vi "Normal mode logic.vi"(9 "Elevator states array":T1[](array[typedef]), 11 "Floors to serve":cluster{"H call":dbl, "Up":bool}[](array[cluster])) -> (1 "Elevator states array out":T1[](array[typedef]), 3 "Floors to serve out":cluster{"H call":dbl, "Up":bool}[](array[cluster]))   [LabVIEW 2019]
uses:
  Type defs/Elevator states.ctl
  Type defs/Elevator position.ctl
  Type defs/Car buttons.ctl
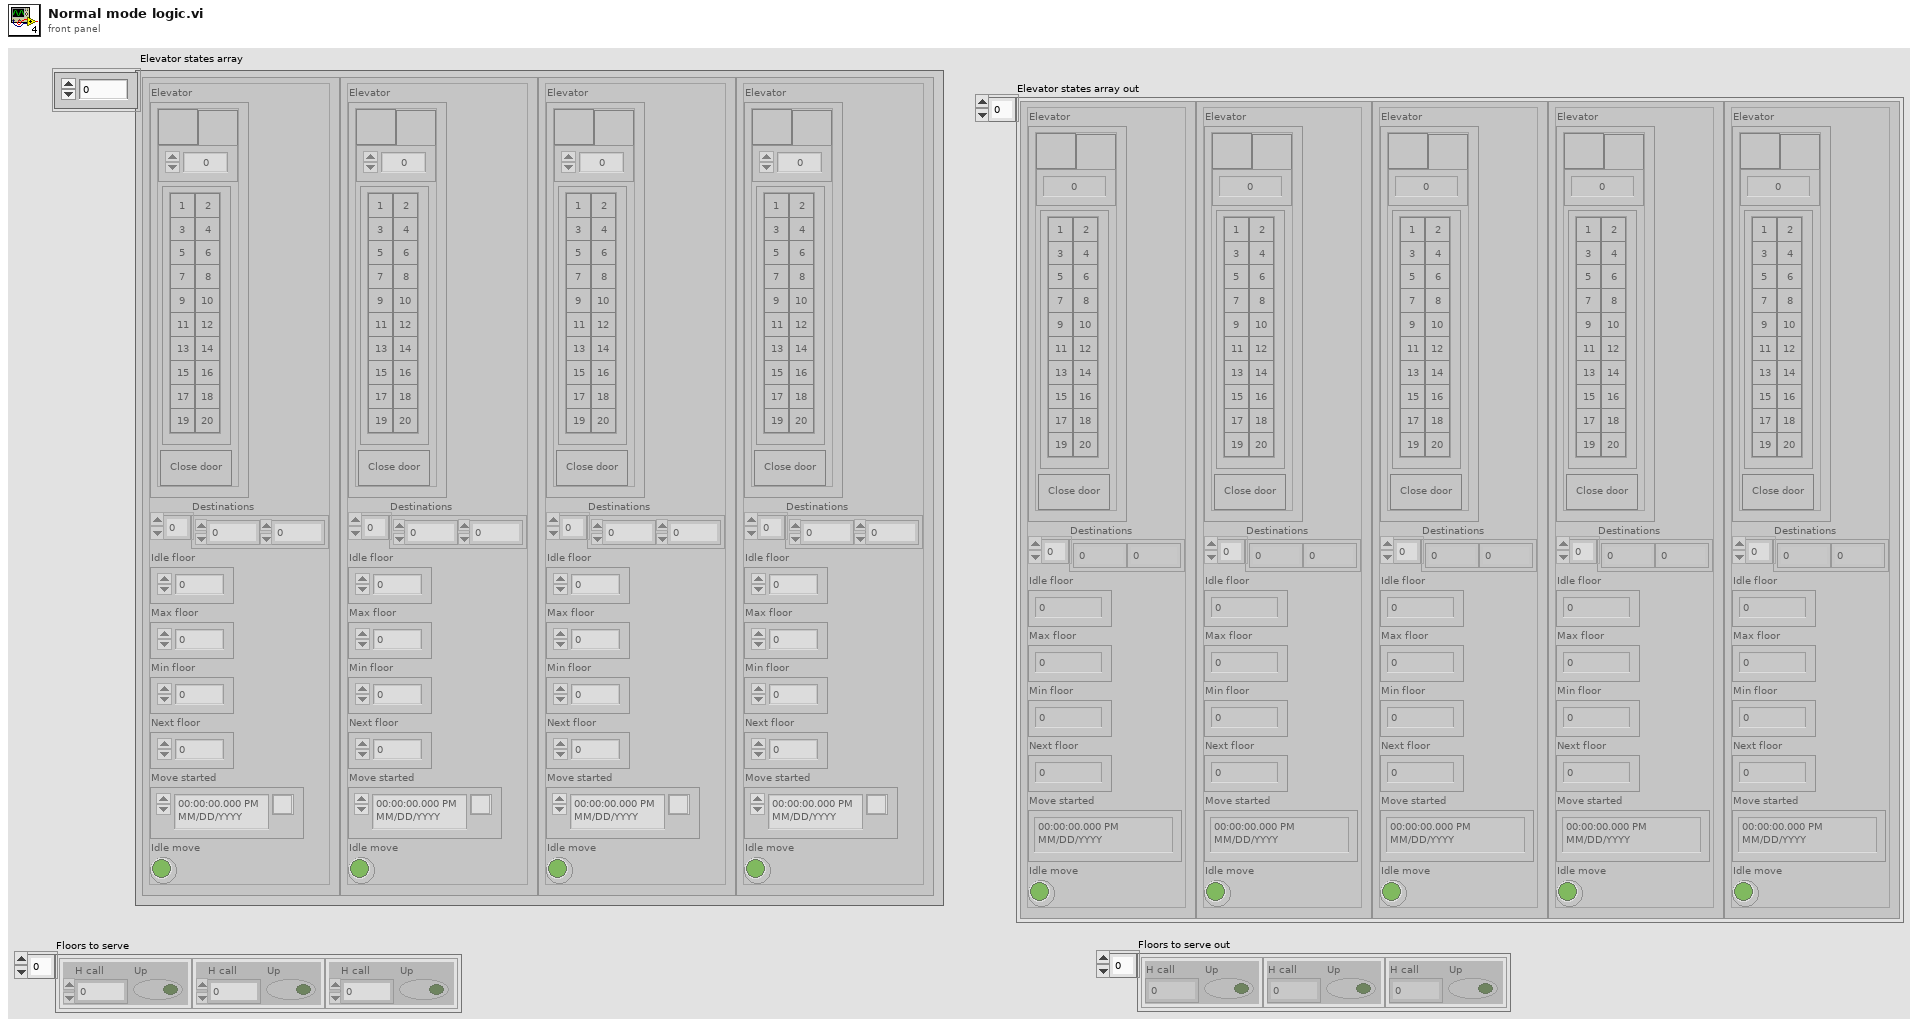
[diagram p1: front panel]
types:
  T1 = typedef "Elevator states.ctl" = cluster{"Elevator":T2, "Destinations":i32[], "Idle floor":u16, "Max floor":u16, "Min floor":u16, "Next floor":u16, "Move started":timestamp, "Idle move":bool}
  T2 = typedef "Elevator position.ctl" = cluster{"Up Button":bool, "Current floor":u16, "Down Button":bool, "Car":T3, "Close door":bool}
  T3 = typedef "Car buttons.ctl" = cluster{"Blank Button":bool, "Blank Button 2":bool, "Blank Button 3":bool, "Blank Button 4":bool, "Blank Button 5":bool, "Blank Button 6":bool, "Blank Button 7":bool, "Blank Button 8":bool, "Blank Button 9":bool, "Blank Button 10":bool, "Blank Button 11":bool, "Blank Button 12":bool, "Blank Button 13":bool, "Blank Button 14":bool, "Blank Button 15":bool, "Blank Button 16":bool, "Blank Button 17":bool, "Blank Button 18":bool, "Blank Button 19":bool, "Blank Button 20":bool}
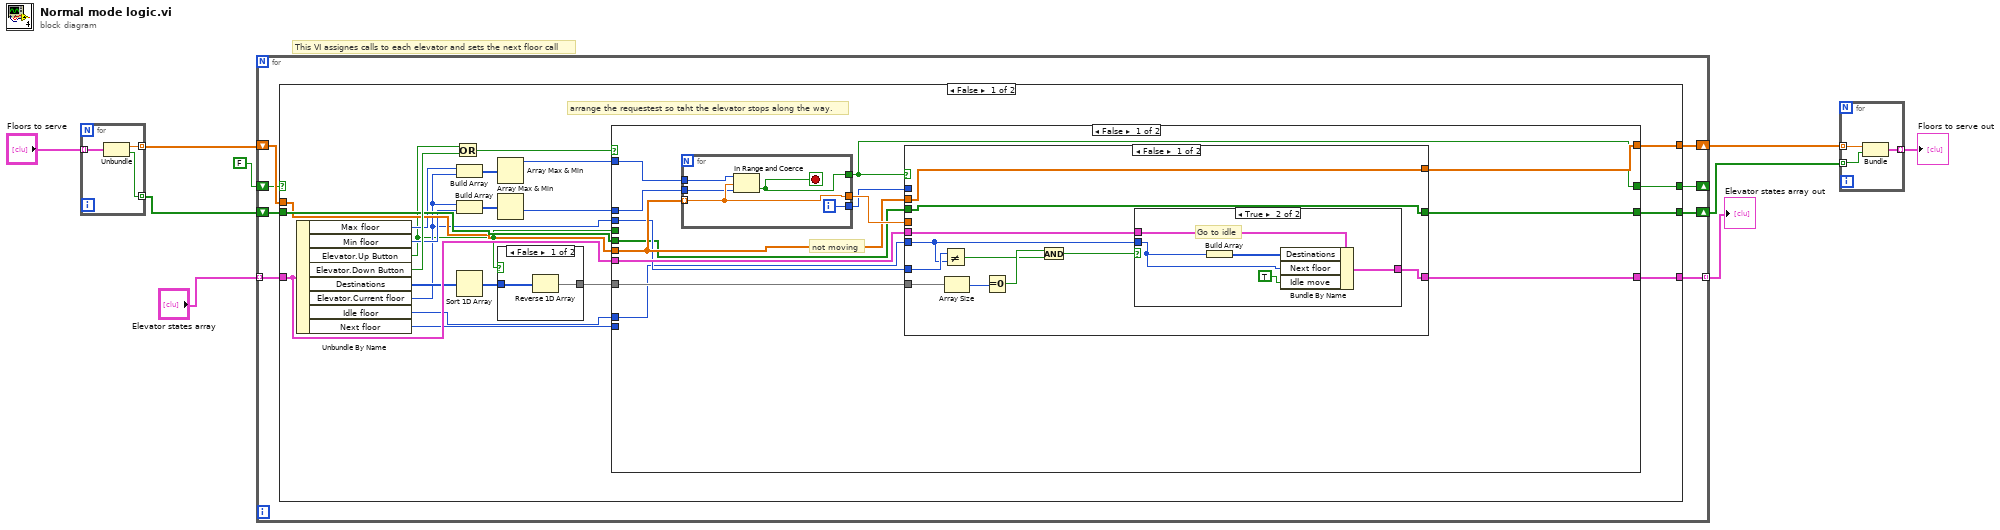
[diagram p0: block diagram]
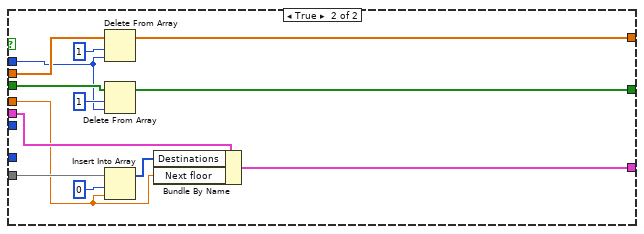
[diagram p4: hidden frame]
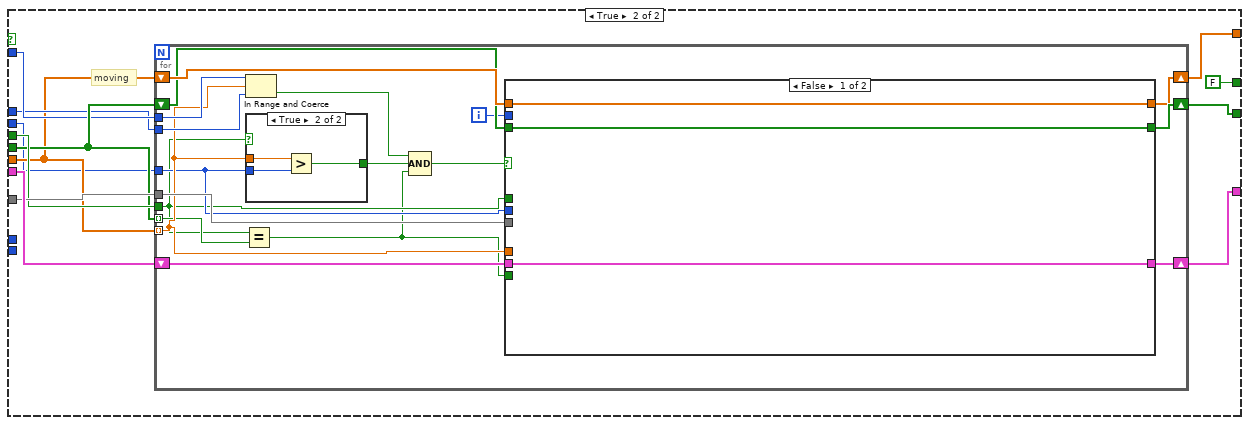
[diagram p5: hidden frame]
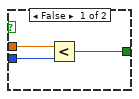
[diagram p6: hidden frame]
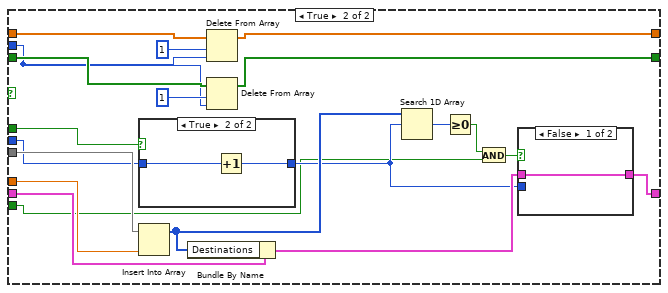
[diagram p7: hidden frame]
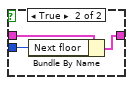
[diagram p8: hidden frame]
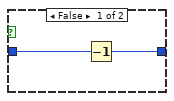
[diagram p9: hidden frame]
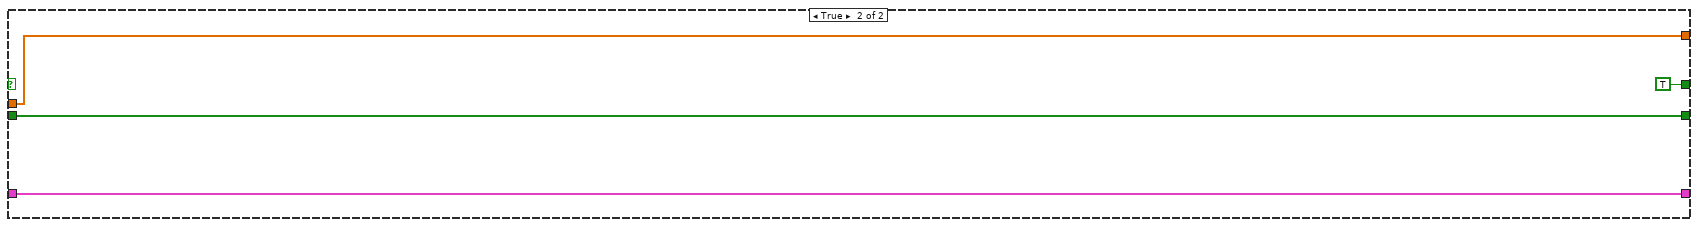
[diagram p10: hidden frame]
diagram:
  # "This VI assignes calls to each elevator and sets the next floor call"
  n1 = for {
    tunnel: "Floors to serve" -> [w12] mode=indexing
    tunnel: [w11] -> w6 mode=indexing
    tunnel: [w10] -> w3 mode=indexing
    n2 = Unbundle(w12) -> ("H call"=w11:dbl, "Up"=w10:bool)
  }
  n3 = for {
    tunnel: "Elevator states array" -> [w20] mode=indexing
    shift-right: [w19] -> w5
    shift-left: w6 -> [w15]
    tunnel: [w18] -> w8 mode=indexing
    shift-right: [w16] -> w2
    shift-left: w3 -> [w17]
    shift-right: [w14] -> _
    shift-left: FALSE -> [w13]
    n4 = case shown="False" w13 {
      tunnel: w20 -> [w40 w164]
      tunnel: [w39 w165] -> w19
      tunnel: [w38 w164] -> w18
      tunnel: w17 -> [w35 w163]
      tunnel: [w34 w163] -> w16
      tunnel: w15 -> [w30 w165]
      tunnel: [w22 TRUE] -> w14
      frame False {
        # "arrange the requestest so taht the elevator stops along the way."
        n5 = Unbundle By Name(w40) -> ("Max floor"=w29:u16, "Min floor"=w26:u16, "Elevator.Up Button"=w21:bool, "Elevator.Down Button"=w42:bool, "Destinations"=w33:i32[], "Elevator.Current floor"=w25:u16, "Idle floor"=w37:u16, "Next floor"=w36:u16)
        n6 = Or(x=w21, y=w42) -> (x .or. y?=w41:bool)
        n7 = Build Array(w29, w25) -> (w28:u16[])
        n8 = Build Array(w25, w26) -> (w24:u16[])
        n9 = Sort 1D Array(array=w33) -> (sorted array=w31:i32[])
        n10 = Array Max & Min(array=w28) -> (max value=w27:u16)  [unwired: 3 out]
        n11 = Array Max & Min(array=w24) -> (min value=w23:u16)  [unwired: 3 out]
        n12 = case shown="False" w21 {
          tunnel: [w44 w45] -> w32
          tunnel: w31 -> [w43 w45]
          frame False {
            n13 = Reverse 1D Array(array=w43) -> (reversed array=w44:i32[])
          }
          frame True {
          }
        }
        n14 = case shown="False" w41 {
          tunnel: w30 -> [w55 w97]
          tunnel: w40 -> [w59 w106]
          tunnel: w32 -> [w58 w105]
          tunnel: [w53 w103] -> w39
          tunnel: [w56 w104] -> w38
          tunnel: w27 -> [w52 w99]
          tunnel: w23 -> [w51 w98]
          tunnel: w25 -> [w50 w95]
          tunnel: w37 -> [w49 _]
          tunnel: w21 -> [_ w101]
          tunnel: w36 -> [_ _]
          tunnel: w35 -> [w48 w100]
          tunnel: [w47 w102] -> w34
          tunnel: [w46 FALSE] -> w22
          frame False {
            # "not moving"
            n15 = for {
              tunnel: w55 -> [w64] mode=indexing
              tunnel: [w60] -> w46
              tunnel: [w64] -> w57
              tunnel: [w63] -> w54
              tunnel: w52 -> [w62]
              tunnel: w51 -> [w61]
              i -> [w63]
              stop <- w60 stop-if-true
              n16 = In Range and Coerce(upper limit=w62, x=w64, lower limit=w61) -> (In Range?=w60:bool)  [unwired: 1 out]
            }
            n17 = case shown="False" w46 {
              tunnel: w59 -> [w68 w94]
              tunnel: w58 -> [w74 w93]
              tunnel: w57 -> [_ w87]
              tunnel: [w67 w91] -> w56
              tunnel: w55 -> [w75 w89]
              tunnel: w54 -> [_ w82]
              tunnel: [w75 w88] -> w53
              tunnel: w50 -> [w72 _]
              tunnel: w49 -> [w66 _]
              tunnel: w48 -> [w65 w84]
              tunnel: [w65 w83] -> w47
              frame False {
                n18 = Not Equal?(x=w72, y=w66) -> (x != y?=w70:bool)
                n19 = Array Size(array=w74) -> (size(s)=w73:i32)
                n20 = Equal To 0?(x=w73) -> (x = 0?=w71:bool)
                n21 = And(x=w71, y=w70) -> (x .and. y?=w69:bool)
                n22 = case shown="True" w69 {
                  tunnel: w68 -> [w76 w81]
                  tunnel: [w76 w80] -> w67
                  tunnel: w66 -> [_ w78]
                  frame False {
                    # "Already at idle"
                  }
                  frame True {
                    # "Go to idle"
                    n23 = Build Array(w78) -> (w79:u16[])
                    n24 = Bundle By Name(cluster=w81, "Destinations"=w79, "Next floor"=w78, "Idle move"=TRUE) -> (w80:T1)
                  }
                }
              }
              frame True {
                n25 = Delete From Array(array=w89, length=1, index=w82) -> (array with subset deleted=w88:dbl[])  [unwired: 1 out]
                n26 = Delete From Array(array=w84, length=1, index=w82) -> (array with subset deleted=w83:bool[])  [unwired: 1 out]
                n27 = Insert Into Array(array=w93, index=0, new element=w87) -> (w92:i32[])
                n28 = Bundle By Name(cluster=w94, "Destinations"=w92, "Next floor"=w87) -> (w91:T1)
              }
            }
          }
          frame True {
            # "moving"
            n29 = for {
              tunnel: w105 -> [w123]
              shift-right: [w121] -> w104
              shift-left: w106 -> [w124]
              shift-right: [w120] -> w102
              shift-left: w100 -> [w119]
              shift-right: [w118] -> w103
              shift-left: w97 -> [w122]
              tunnel: w101 -> [w108]
              tunnel: w100 -> [w109] mode=indexing
              tunnel: w99 -> [w116]
              tunnel: w98 -> [w115]
              tunnel: w97 -> [w112] mode=indexing
              tunnel: w95 -> [w111]
              i -> [w117]
              n30 = Equal?(x=w108, y=w109) -> (x = y?=w107:bool)
              n31 = In Range and Coerce(upper limit=w116, x=w112, lower limit=w115) -> (In Range?=w114:bool)  [unwired: 1 out]
              n32 = case shown="True" w108 {
                tunnel: w112 -> [w126 w130]
                tunnel: w111 -> [w127 w129]
                tunnel: [w125 w128] -> w110
                frame False {
                  n33 = Less?(x=w126, y=w127) -> (x < y?=w125:bool)
                }
                frame True {
                  n34 = Greater?(x=w130, y=w129) -> (0:w128:bool)
                }
              }
              n35 = Compound Arithmetic op=AND(w114, w110, w107) -> (w113:bool)
              n36 = case shown="False" w113 {
                tunnel: w124 -> [w133 w153]
                tunnel: w123 -> [_ w152]
                tunnel: w122 -> [w132 w151]
                tunnel: [w132 w149] -> w118
                tunnel: [w133 w137] -> w121
                tunnel: w119 -> [w131 w147]
                tunnel: [w131 w146] -> w120
                tunnel: w108 -> [_ w143]
                tunnel: w117 -> [_ w145]
                tunnel: w112 -> [_ w144]
                tunnel: w111 -> [_ w142]
                tunnel: w107 -> [_ w135]
                frame False {
                }
                frame True {
                  n37 = case shown="True" w143 {
                    tunnel: w142 -> [w159 w161]
                    tunnel: [w158 w160] -> w136
                    frame False {
                      n38 = Decrement(x=w159) -> (x-1=w158:u16)
                    }
                    frame True {
                      n39 = Increment(x=w161) -> (x+1=w160:u16)
                    }
                  }
                  n40 = Insert Into Array(array=w152, new element=w144) -> (w141:i32[])  [unwired: 1 in]
                  n41 = Bundle By Name(cluster=w153, "Destinations"=w141) -> (w138:T1)
                  n42 = Delete From Array(array=w151, length=1, index=w145) -> (array with subset deleted=w149:dbl[])  [unwired: 1 out]
                  n43 = Delete From Array(array=w147, length=1, index=w145) -> (array with subset deleted=w146:bool[])  [unwired: 1 out]
                  n44 = Search 1D Array(1D array=w141, element=w136) -> (index of element=w140:i32)  [unwired: 1 in]
                  n45 = Greater Or Equal To 0?(x=w140) -> (x >= 0?=w139:bool)
                  n46 = And(x=w139, y=w135) -> (x .and. y?=w134:bool)
                  n47 = case shown="False" w134 {
                    tunnel: w138 -> [w154 w157]
                    tunnel: [w154 w156] -> w137
                    tunnel: w136 -> [_ w155]
                    frame False {
                    }
                    frame True {
                      n48 = Bundle By Name(cluster=w157, "Next floor"=w155) -> (w156:T1)
                    }
                  }
                }
              }
            }
          }
        }
      }
      frame True {
      }
    }
  }
  "Elevator states array out" <- w8
  n49 = for {
    tunnel: w5 -> [w168] mode=indexing
    tunnel: [w167] -> w4 mode=indexing
    tunnel: w2 -> [w166] mode=indexing
    n50 = Bundle("H call"=w168, "Up"=w166) -> (w167:cluster{"H call":dbl, "Up":bool})  [unwired: 1 in]
  }
  "Floors to serve out" <- w4
